vi "MPDSnC Send Command.vi"(0 "VISA Ref":refnum<visa-resource-name>, 2 "Wait for Reply?":bool=TRUE, 7 "Error In":errorcluster, 11 "Command":string) -> (4 "VISA Ref Out":refnum<visa-resource-name>, 8 "Error Out":errorcluster, 15 "Response":string)   [LabVIEW 2016]
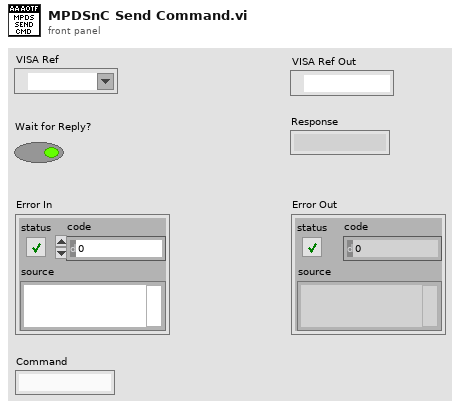
[diagram p1: front panel]
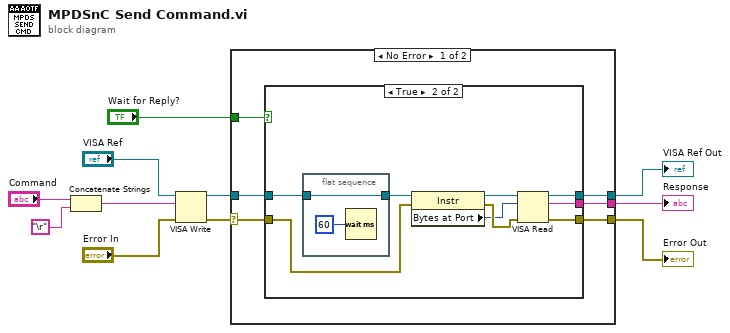
[diagram p0: block diagram]
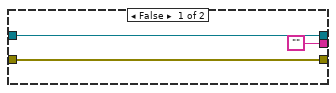
[diagram p2: hidden frame]
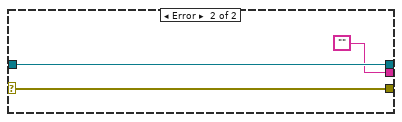
[diagram p3: hidden frame]
diagram:
  n1 = Concatenate Strings("Command", "\r") -> (w2:string)
  n2 = VISA Write(VISA resource name="VISA Ref", write buffer=w2, error in (no error)="Error In") -> (VISA resource name out=w11:refnum<visa-resource-name>, error out=w1:errorcluster)  [unwired: 1 out]
  n3 = case shown="No Error" w1 {
    selector: w1 -> [w12 w33]
    tunnel: w11 -> [w17 w34]
    tunnel: [w16 w34] -> w9
    tunnel: [w15 w33] -> w8
    tunnel: [w14 ""] -> w6
    tunnel: "Wait for Reply?" -> [w13 _]
    frame No Error {
      n4 = case shown="True" w13 {
        tunnel: w17 -> [w20 w25]
        tunnel: w12 -> [w19 w24]
        tunnel: [w20 w23] -> w16
        tunnel: [w19 w22] -> w15
        tunnel: ["" w21] -> w14
        frame False {
        }
        frame True {
          n5 = flat-sequence {
            tunnel: [w30] -> w28
            tunnel: w25 -> [w30]
            frame #0 {
              n6 = Wait (ms)(milliseconds to wait=u32 60) -> ()  [unwired: 1 out]
            }
          }
          n7 = property class="Instr"(reference=w28, error in=w24) -> (reference out=w26:refnum<visa-resource-name>, error out=w29:errorcluster, "Bytes at Port"=w27:u32)
          n8 = VISA Read(VISA resource name=w26, byte count=w27, error in (no error)=w29) -> (VISA resource name out=w23:refnum<visa-resource-name>, read buffer=w21:string, error out=w22:errorcluster)  [unwired: 1 out]
        }
      }
    }
    frame Error {
    }
  }
  "Response" <- w6
  "VISA Ref Out" <- w9
  "Error Out" <- w8
